vi "Form Groups.vi"(10 "Max Size in":i32, 11 "Array in":T1[](array[typedef]) {"Mapping"."VS Reference" format="%.0x"}) -> (3 "Array out":T7[](array[typedef]) {"Channel Data"."Mapping"."VS Reference" format="%.0x"})   [LabVIEW 2021, in "Modbus Master System Explorer.lvlib"]
uses:
  Modbus Master System Explorer.lvlib
  Engine/SubVIs/Bulk Data Access.ctl
  Modbus Type.ctl
  Shared/Controls/Data Model/Channel.ctl
  <vilib>/NI VeriStand/Custom Device API/Custom Device Channel Type.ctl
  Shared/Controls/Data Model/Mapping.ctl
  Shared/Controls/Data Model/DataType.ctl
  <vilib>/NI VeriStand/Custom Device API/Custom Device Item Ref.ctl
  <vilib>/NI VeriStand/Custom Device API/Custom Device API.lvlib
  Shared/Modbus Master Shared.lvlib
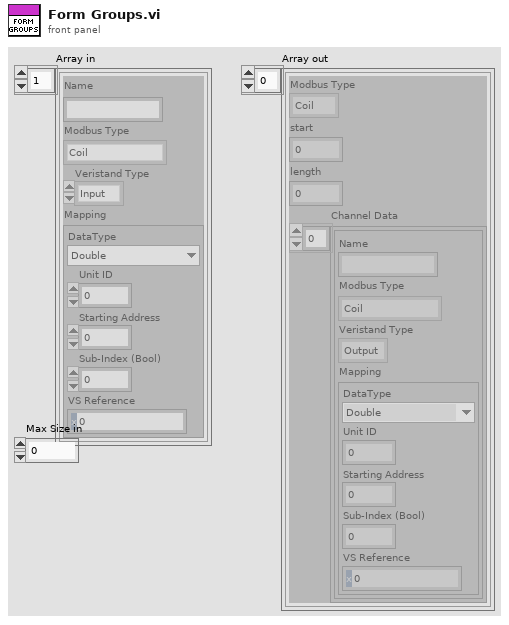
[diagram p1: front panel]
types:
  T1 = typedef "Modbus Master Shared.lvlib/Channel.ctl" = cluster{"Name":string, "Modbus Type":T2, "Veristand Type":T3, "Mapping":T4}
  T2 = typedef "Modbus Master Shared.lvlib/Modbus Type.ctl" = enum16{"Coil", "Discrete Input", "Holding Register", "Input Register"}
  T3 = typedef "Custom Device API.lvlib/Custom Device Channel Type.ctl" = enum16{"Input", "Output"}
  T4 = typedef "Modbus Master Shared.lvlib/Mapping.ctl" = cluster{"DataType":T5, "Unit ID":u8, "Starting Address":u16, "Sub-Index (Bool)":u16, "VS Reference":T6}
  T5 = typedef "Modbus Master Shared.lvlib/DataType.ctl" = enum16{"Double", "Single", "I64", "I32", "I16", "I8", "U64", "U32", "U16", "U8", "Boolean"}
  T6 = typedef "Custom Device API.lvlib/Custom Device Item Ref.ctl" = u64
  T7 = typedef "Modbus Master Shared.lvlib/Bulk Data Access.ctl" = cluster{"Modbus Type":T2, "start":u16, "length":u16, "Channel Data":T1[]}
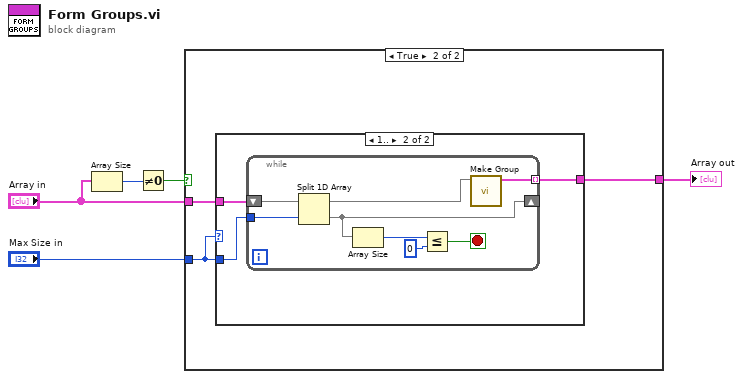
[diagram p0: block diagram]
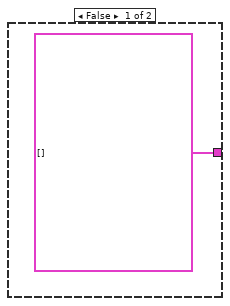
[diagram p2: hidden frame]
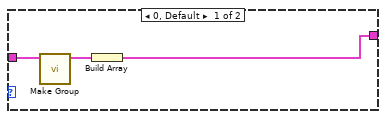
[diagram p3: hidden frame]
diagram:
  n1 = Array Size(array="Array in") -> (size(s)=w2:i32)
  n2 = Not Equal To 0?(x=w2) -> (x != 0?=w1:bool)
  n3 = case shown="True" w1 {
    tunnel: [T7[] [] w9] -> w5
    tunnel: "Max Size in" -> [_ w8]
    tunnel: "Array in" -> [_ w7]
    frame False {
    }
    frame True {
      n4 = case shown="1.." w8 {
        tunnel: [w10 w13] -> w9
        tunnel: w7 -> [w12 w15]
        tunnel: w8 -> [_ w14]
        frame 0, Default {
          n5 = call "Make Group.vi"("Array in"=w12) -> ("Group"=w11:T7)  [unwired: 10 in]
          n6 = Build Array(w11) -> (w10:T7[])
        }
        frame 1.. {
          n7 = while {
            tunnel: w14 -> [w21]
            shift-right: [w20] -> _
            shift-left: w15 -> [w23]
            tunnel: [w16] -> w13 mode=indexing
            stop <- w18 stop-if-true
            n8 = Split 1D Array(array=w23, index=w21) -> (first subarray=w17:T1[], second subarray=w20:T1[])
            n9 = Array Size(array=w20) -> (size(s)=w22:i32)
            n10 = Less Or Equal?(x=w22, y=0) -> (x <= y?=w18:bool)
            n11 = call "Make Group.vi"("Array in"=w17) -> ("Group"=w16:T7)  [unwired: 10 in]
          }
        }
      }
    }
  }
  "Array out" <- w5
